vi "EX - Execute a program.vi"(1 "Run Stored\n Program #":i8=1 min=1 max=6 step=1, 2 "error in":errorcluster, 3 "# of times\nto execute":dbl format="%.2f", 4 "Address / Port":i16=1 min=1 max=31 step=1) -> (0 "error out":errorcluster)   [LabVIEW 2014]
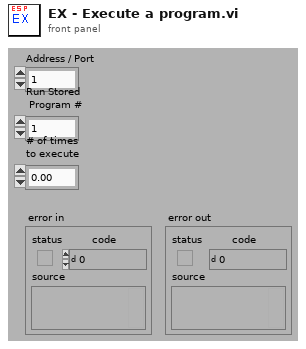
[diagram p1: front panel]
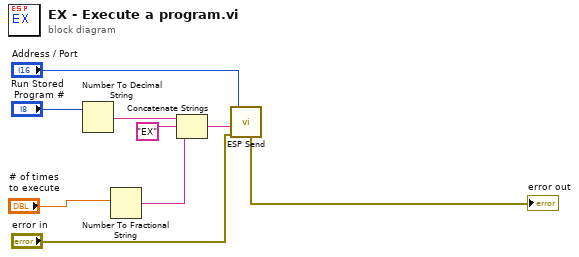
[diagram p0: block diagram]
diagram:
  n1 = Number To Decimal String(number="Run Stored\n Program #") -> (decimal integer string=w8:string)  [unwired: 1 in]
  n2 = Number To Fractional String(number="# of times\nto execute") -> (F-format string=w1:string)  [unwired: 3 in]
  n3 = Concatenate Strings(w8, "EX" ("Substring"), w1) -> (w6:string)
  n4 = call "ESP Send.vi"("Address / Port"="Address / Port", "Command String"=w6, "error in"="error in") -> ("error out"=→"error out":errorcluster)  [unwired: 5 in]
